vi "str to datetime.vi"(2 "String":string) -> (6 "Time Stamp":timestamp)   [LabVIEW 2014, in "OPCUA XML.lvlib"]
uses:
  OPCUA XML.lvlib
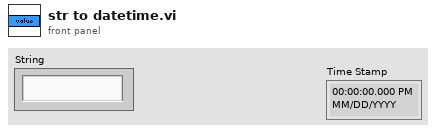
[diagram p1: front panel]
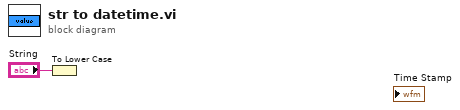
[diagram p0: block diagram]
diagram:
  n1 = To Lower Case(string="String") -> ()  [unwired: 1 out]
